vi "Create Waveform Channel.vi"(8 "error in (no error)":errorcluster, 10 "Bitfile Name":string, 11 "Item Ref in":T1 format="%.0x") -> (0 "error out":errorcluster)   [LabVIEW 2020, in "FPGA Addon System Explorer.lvlib"]
uses:
  FPGA Addon System Explorer.lvlib
  <vilib>/NI VeriStand/Custom Device API/Custom Device API.lvlib
  Addon Shared/SubVIs/Constants.vi
  Addon Shared/FPGA Addon Shared.lvlib
  <vilib>/NI VeriStand/Custom Device API/Custom Device Channel Type.ctl
  <vilib>/NI VeriStand/Custom Device API/Custom Device Channel.ctl
  <vilib>/NI VeriStand/Custom Device API/Custom Device Item Ref.ctl
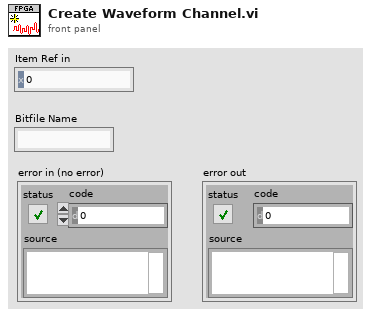
[diagram p1: front panel]
types:
  T1 = typedef "Custom Device API.lvlib/Custom Device Item Ref.ctl" = u64
  T2 = typedef "Custom Device API.lvlib/Custom Device Channel.ctl" = cluster{"Type":T3, "Units":string, "Default Value":dbl, "Faultable":bool, "Scalable":bool}
  T3 = typedef "Custom Device API.lvlib/Custom Device Channel Type.ctl" = enum16{"Input", "Output"}
  T4 = enum32{"invalid app kind", "Development System", "Run Time System", "Student Edition", "Embedded LabVIEW", "Evaluation", "Custom"}
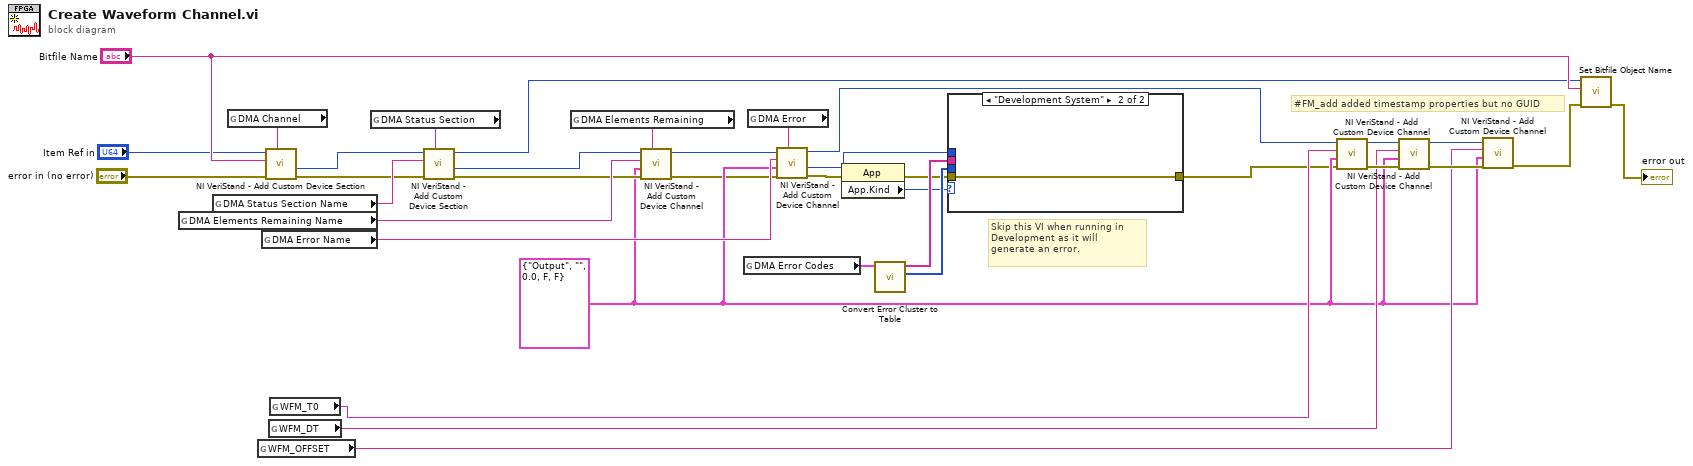
[diagram p0: block diagram]
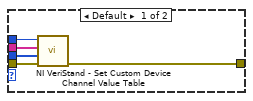
[diagram p2: hidden frame]
diagram:
  w6 = T2 {"Type"=enum."Output", "Units"="", "Default Value"=0.0, "Faultable"=FALSE, "Scalable"=FALSE} ("Channel")
  # "#FM_add added timestamp properties but no GUID"
  # "Skip this VI when running in Development as it will generate an error."
  n1 = global read "Constants.vi" "DMA Elements Remaining Name"() -> (w25:string)
  n2 = global read "Constants.vi" "DMA Status Section Name"() -> (w28:string)
  n3 = global read "Constants.vi" "DMA Channel"() -> (w19:string)
  n4 = global read "Constants.vi" "WFM_OFFSET"() -> (w7:string)
  n5 = global read "Constants.vi" "DMA Error Name"() -> (w26:string)
  n6 = call <vilib>:"NI VeriStand - Add Custom Device Section.vi"("GUID (Default Section)"=w19, "error in (no error)"="error in (no error)", "Section Name"="Bitfile Name", "Parent Ref in"="Item Ref in") -> ("error out"=w20:errorcluster, "Section Ptr"=w21:T1)  [unwired: 4 in, 2 out]
  n7 = global read "Constants.vi" "WFM_DT"() -> (w8:string)
  n8 = global read "Constants.vi" "WFM_T0"() -> (w9:string)
  n9 = global read "Constants.vi" "DMA Status Section"() -> (w29:string)
  n10 = call <vilib>:"NI VeriStand - Add Custom Device Section.vi"("GUID (Default Section)"=w29, "error in (no error)"=w20, "Section Name"=w28, "Parent Ref in"=w21) -> ("error out"=w23:errorcluster, "Section Ptr"=w22:T1, "Parent Ref out"=w34:T1)  [unwired: 4 in, 1 out]
  n11 = global read "Constants.vi" "DMA Elements Remaining"() -> (w24:string)
  n12 = call <vilib>:"NI VeriStand - Add Custom Device Channel.vi"("GUID (Default Channel)"=w24, "error in (no error)"=w23, "Channel"=w6, "Channel Name"=w25, "Parent Ref in"=w22) -> ("error out"=w4:errorcluster, "Parent Ref out"=w5:T1)  [unwired: 3 in, 2 out]
  n13 = global read "Constants.vi" "DMA Error Codes"() -> (w30:cluster{"number":i32, "trimmed string":string}[])
  n14 = global read "Constants.vi" "DMA Error"() -> (w27:string)
  n15 = call <vilib>:"NI VeriStand - Add Custom Device Channel.vi"("GUID (Default Channel)"=w27, "error in (no error)"=w4, "Channel"=w6, "Channel Name"=w26, "Parent Ref in"=w5) -> ("error out"=w16:errorcluster, "Channel Ref"=w31:T1, "Parent Ref out"=w3:T1)  [unwired: 3 in, 1 out]
  n16 = property class="App"(error in=w16) -> (error out=w15:errorcluster, "App.Kind"=w14:T4)  [unwired: 1 in, 1 out]
  n17 = call "Convert Error Cluster to Table.vi"("Error Codes"=w30) -> ("Code"=w33:i32[], "String"=w32:string[])  [unwired: 9 in]
  n18 = case shown="\"Development System\"" w14 {
    tunnel: [w41 w42] -> w1
    tunnel: w33 -> [w40 _]
    tunnel: w32 -> [w39 _]
    tunnel: w31 -> [w38 _]
    tunnel: w15 -> [w37 w42]
    frame Default {
      n19 = call <vilib>:"NI VeriStand - Set Custom Device Channel Value Table.vi"("error in (no error)"=w37, "Values"=w40, "Names"=w39, "Channel Ref in"=w38) -> ("error out"=w41:errorcluster)  [unwired: 6 in, 1 out]
    }
    frame "Development System" {
    }
  }
  n20 = call <vilib>:"NI VeriStand - Add Custom Device Channel.vi"("error in (no error)"=w1, "Channel"=w6, "Channel Name"=w9, "Parent Ref in"=w3) -> ("error out"=w12:errorcluster, "Parent Ref out"=w13:T1)  [unwired: 4 in, 2 out]
  n21 = call <vilib>:"NI VeriStand - Add Custom Device Channel.vi"("error in (no error)"=w12, "Channel"=w6, "Channel Name"=w8, "Parent Ref in"=w13) -> ("error out"=w10:errorcluster, "Parent Ref out"=w11:T1)  [unwired: 4 in, 2 out]
  n22 = call <vilib>:"NI VeriStand - Add Custom Device Channel.vi"("error in (no error)"=w10, "Channel"=w6, "Channel Name"=w7, "Parent Ref in"=w11) -> ("error out"=w2:errorcluster)  [unwired: 4 in, 3 out]
  n23 = call "Set Bitfile Object Name.vi"("error in (no error)"=w2, "Name"="Bitfile Name", "Channel Ref"=w34) -> ("error out"=→"error out":errorcluster)  [unwired: 8 in]
